vi "[SubVI]Data_Write.vi"(1 "1D data":dbl[](array[numeric]), 2 "Saving File Name":string) -> ()   [LabVIEW 2017]
uses:
  <vilib>/Utility/file.llb/Write Delimited Spreadsheet (DBL).vi
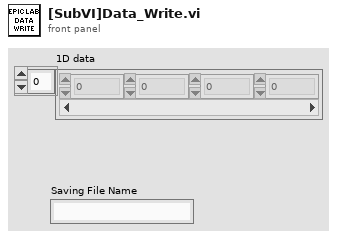
[diagram p1: front panel]
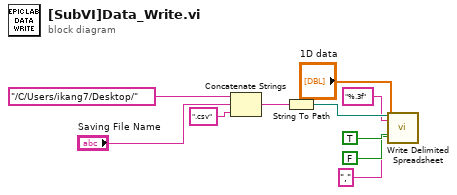
[diagram p0: block diagram]
diagram:
  n1 = Concatenate Strings("/C/Users/ikang7/Desktop/", "Saving File Name", ".csv") -> (w4:string)
  n2 = String To Path(string=w4) -> (path=w8:path)
  n3 = call-poly <vilib>:"Write Delimited Spreadsheet.vi"("file path (dialog if empty)"=w8, "format (%.3f)"="%.3f", "1D data"="1D data", "append to file? (new file:F)"=TRUE, "transpose? (no:F)"=FALSE, "delimiter (\\t)"="," ("delimiter (\\t)")) -> ()  [unwired: 8 in, 2 out]
